vi "Dispatch_FindOrFilterOnName.vi"(8 "error in":errorcluster, 9 "function path":path, 10 "Data Tree in":refnum<vi>, 11 "SubPanel in":refnum<vi>) -> (0 "error out":errorcluster, 2 "Data Tree out":refnum<vi>, 3 "SubPanel out":refnum<vi>)   [LabVIEW 2013, in "FindName Task_Manager.lvlib"]
doc: "Invokes the specified function VI, ACBR style."
uses:
  FindName Task_Manager.lvlib
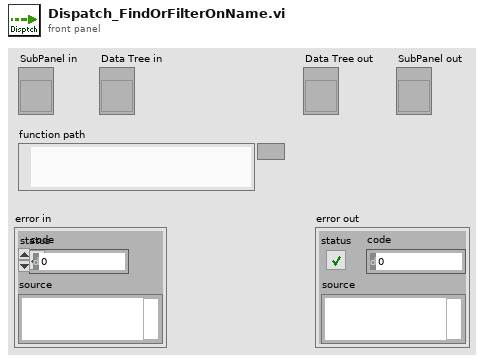
[diagram p1: front panel]
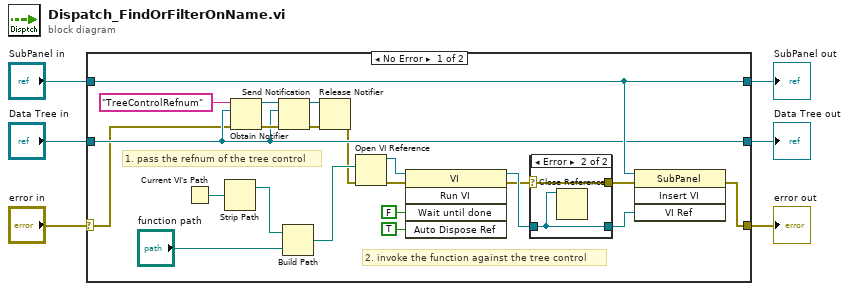
[diagram p0: block diagram]
diagram:
  n1 = case shown="No Error" "error in" {
    selector: "error in" -> [w7 w35]
    tunnel: [w20 w35] -> w6
    tunnel: "SubPanel in" -> [w12 w34]
    tunnel: "Data Tree in" -> [w11 w33]
    tunnel: [w12 w34] -> w2
    tunnel: [w11 w33] -> w1
    frame No Error {
      # "2. invoke the function against the tree control"
      # "1. pass the refnum of the tree control"
      n2 = Current VI's Path() -> (path=w23:path)
      n3 = Strip Path(path=w23) -> (stripped path=w10:path)  [unwired: 1 out]
      n4 = Obtain Notifier(name (unnamed)="TreeControlRefnum", notification data type=w11, error in (no error)=w7) -> (notifier out=w13:refnum<notifier>, error out=w14:errorcluster)  [unwired: 1 in, 1 out]
      n5 = Send Notification(notification=w11, notifier=w13, error in (no error)=w14) -> (notifier out=w8:refnum<notifier>, error out=w16:errorcluster)
      n6 = Build Path(base path=w10, name or relative path="function path") -> (appended path=w22:path)
      n7 = Release Notifier(notifier=w8, error in (no error)=w16) -> (error out=w9:errorcluster)  [unwired: 1 in, 2 out]
      n8 = Open VI Reference(vi path=w22, error in (no error)=w9) -> (vi reference=w17:refnum<vi>, error out=w19:errorcluster)  [unwired: 4 in]
      n9 = invoke class="VI" method="Run VI"(reference=w17, error in=w19, "Wait until done"=FALSE ("Wait Until Done"), "Auto Dispose Ref"=TRUE ("Auto Dispose Reference")) -> (reference out=w25:refnum<vi>, error out=w24:errorcluster)  [unwired: 1 in, 3 out]
      n10 = case shown="Error" w24 {
        selector: w24 -> [w30 w32]
        tunnel: [w30 w32] -> w27
        tunnel: w25 -> [w29 w31]
        tunnel: [w29 w31] -> w26
        frame No Error {
        }
        frame Error {
          n11 = Close Reference(reference=w31) -> ()  [unwired: 1 in, 1 out]
        }
      }
      n12 = invoke on="Invoke Node" class="SubPanel" method="Insert VI"(reference=w12, error in=w27, "VI Ref"=w26) -> (error out=w20:errorcluster)  [unwired: 1 in, 3 out]
    }
    frame Error {
    }
  }
  "error out" <- w6
  "SubPanel out" <- w2
  "Data Tree out" <- w1
